vi "UDP Refresh Communication Settings.vi"(8 "error in (no error)":errorcluster, 10 "UDP UI References":T1, 11 "node References":T2) -> (0 "error out":errorcluster, 2 "UDP UI References out":T1, 3 "node References out":T2)   [LabVIEW 2015, in "E2E Tag Exchange editor node.lvclass"]
uses:
  E2E Tag Exchange editor node.lvclass
  object references.ctl
  <vilib>/NI/DCAF/Tag Editor Core/Configuration Editor/Classes/Engine Parent/Engine Parent Editor Node.lvclass
  implementation specific/UDP/UDP UI References.ctl
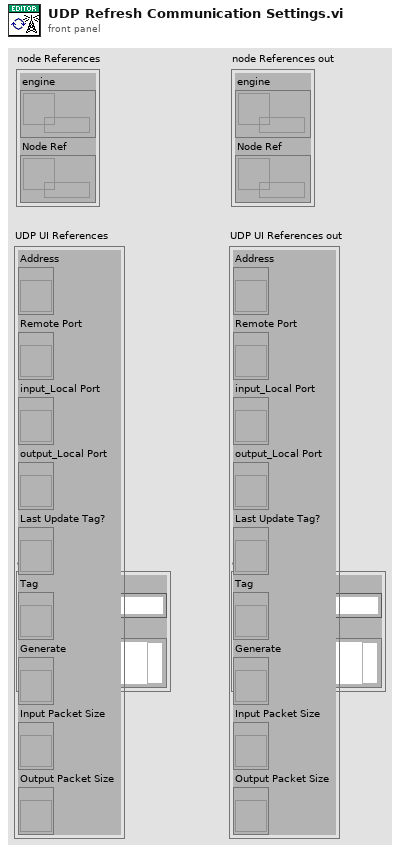
[diagram p1: front panel]
types:
  T1 = typedef "E2E Tag Exchange editor node.lvclass/UDP UI References.ctl" = cluster{"Address":refnum<vi>, "Remote Port":refnum<vi>, "input_Local Port":refnum<vi>, "output_Local Port":refnum<vi>, "Last Update Tag?":refnum<vi>, "Tag":refnum<vi>, "Generate":refnum<vi>, "Input Packet Size":refnum<vi>, "Output Packet Size":refnum<vi>}
  T2 = typedef "E2E Tag Exchange editor node.lvclass/object references.ctl" = cluster{"engine":refnum<data-value>, "Node Ref":refnum<data-value>}
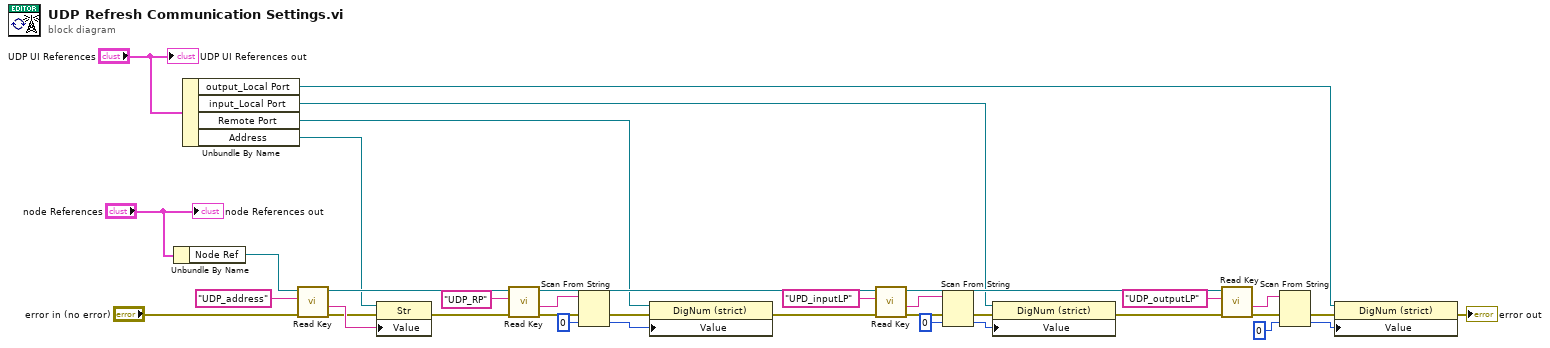
[diagram p0: block diagram]
diagram:
  n1 = Unbundle By Name("node References") -> ("Node Ref"=w8:refnum<data-value>)
  n2 = Unbundle By Name("UDP UI References") -> ("output_Local Port"=w5:refnum<vi>, "input_Local Port"=w4:refnum<vi>, "Remote Port"=w3:refnum<vi>, "Address"=w2:refnum<vi>)
  n3 = call "Read Key.vi"("error in (no error)"="error in (no error)", "Key"="UDP_address", "E2E editor node in"=w8) -> ("error out"=w10:errorcluster, "Value"=w11:string, "E2E editor node out"=w13:refnum<data-value>)  [unwired: 6 in]
  n4 = property class="Str"(reference=w2, error in=w10, "Value"=w11) -> (error out=w12:errorcluster)  [unwired: 1 out]
  n5 = call "Read Key.vi"("error in (no error)"=w12, "Key"="UDP_RP", "E2E editor node in"=w13) -> ("error out"=w15:errorcluster, "Value"=w16:string, "E2E editor node out"=w21:refnum<data-value>)  [unwired: 6 in]
  n6 = Scan From String(input string=w16, error in=w15, default 1=u16 0 ("Remote Port")) -> (error out=w18:errorcluster, output 1=w19:u16)  [unwired: 2 in, 2 out]
  n7 = property class="DigNum (strict)"(reference=w3, error in=w18, "Value"=w19) -> (error out=w20:errorcluster)  [unwired: 1 out]
  n8 = call "Read Key.vi"("error in (no error)"=w20, "Key"="UPD_inputLP", "E2E editor node in"=w21) -> ("error out"=w23:errorcluster, "Value"=w24:string, "E2E editor node out"=w29:refnum<data-value>)  [unwired: 6 in]
  n9 = Scan From String(input string=w24, error in=w23, default 1=u16 0 ("Remote Port")) -> (error out=w26:errorcluster, output 1=w27:u16)  [unwired: 2 in, 2 out]
  n10 = property class="DigNum (strict)"(reference=w4, error in=w26, "Value"=w27) -> (error out=w28:errorcluster)  [unwired: 1 out]
  n11 = call "Read Key.vi"("error in (no error)"=w28, "Key"="UDP_outputLP", "E2E editor node in"=w29) -> ("error out"=w32:errorcluster, "Value"=w33:string)  [unwired: 6 in, 1 out]
  n12 = Scan From String(input string=w33, error in=w32, default 1=u16 0 ("Remote Port")) -> (error out=w34:errorcluster, output 1=w35:u16)  [unwired: 2 in, 2 out]
  n13 = property class="DigNum (strict)"(reference=w5, error in=w34, "Value"=w35) -> (error out=→"error out":errorcluster)  [unwired: 1 out]
  "node References out" <- "node References"
  "UDP UI References out" <- "UDP UI References"
